vi "Wait for Return Message on FIFO Publisher.vi"(8 "error in (no error)":errorcluster, 9 "Timeout (ms)":u32=1000, 11 "CIFChannelMng in":refnum<class "CIFChannelMng.lvclass">) -> (0 "error out":errorcluster, 1 "Timeout":bool, 2 "FIFO Publisher":T1, 3 "CIFChannelMng out":refnum<class "CIFChannelMng.lvclass">)   [LabVIEW 2021, in "CIFChannelMng.lvclass"]
uses:
  CIFChannelMng.lvclass
  OOB/OOB_Tx/Typedef/FIFO Publisher Return.ctl
  typedef/Errors Channel Manager.ctl
  CIFChannelMng.lvclass/CIFChannelMng.ctl
  <vilib>/CIF Foundation/CIF Out of Band Commands/CIFOutOfBand.lvclass/CIFOutOfBand.ctl
  <vilib>/CIF Foundation/CIF Out of Band Commands/Read Commands.vi
  OOB/OOB_Tx/Private/Command Settings.vi
  OOB/OOB_Tx/Private/Read Payload.vi
  <vilib>/CIF Foundation/CIF Utilities/Errors/Append Error Location.vi
  <vilib>/CIF Foundation/CIF Out of Band Commands/Accessors/Read Local OOB Data.vi
  OOB/OOB_Tx/ChnMngOOB_Tx.lvclass
  C:/Program Files/National Instruments/LabVIEW 2021/vi.lib/CIF Foundation/CIF Out of Band Commands/CIFOutOfBand.lvclass
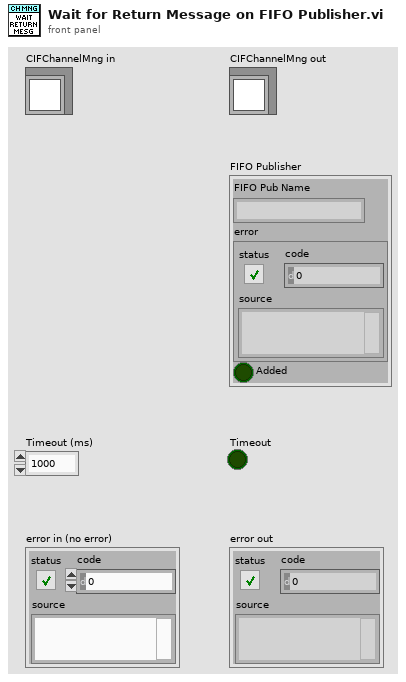
[diagram p1: front panel]
types:
  T1 = typedef "ChnMngOOB_Tx.lvclass/FIFO Publisher Return.ctl" = cluster{"FIFO Pub Name":string, "error":errorcluster, "Added":bool}
  T2 = typedef "CIFChannelMng.lvclass/Errors Channel Manager.ctl" = enum16{"gRPC Server Not Found", "Duplicate Channel", "Missing Channel", "Incorrect Type", "Flatten Error", "Unflatten Data", "Channel Length", "Plugin Connection", "gRPC Server Connection", "FIFO Unflatten", "Required Override", "Remove Not Found", "Skipped due to warning", "Timeout FIFO Pub"}
  T3 = typedef "ChnMngOOB_Tx.lvclass/OOB Core Commands.ctl" = enum8{"Channel List", "New FIFO Pub"}
  T4 = typedef "CIFChannelMng.lvclass/Channel List for OOB.ctl" = cluster{"Name":string, "Direction":T5, "Type":string, "Connected?":bool, "Connected Name":string, "Custom Config Data":u8[], "Forced?":bool, "Multi-Writer":bool}
  T5 = typedef "CIFChannels.lvclass/Direction.ctl" = enum16{"Publisher", "Subscriber"}
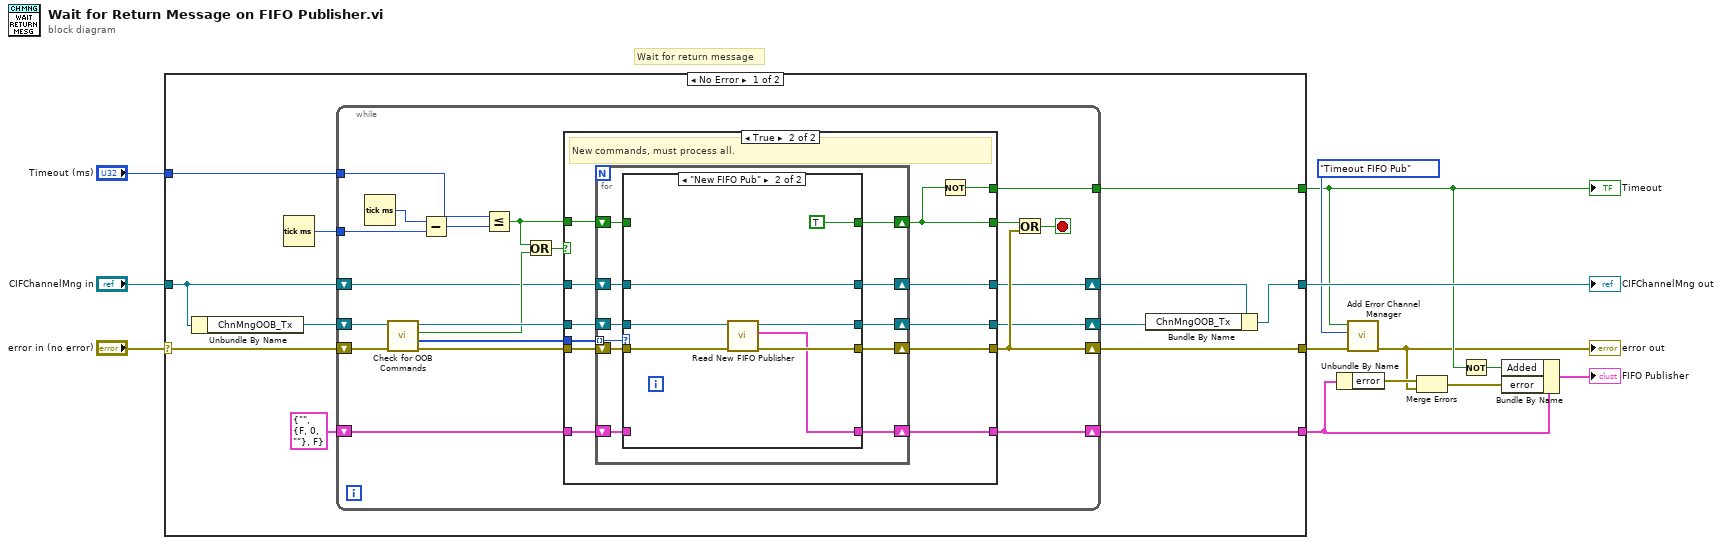
[diagram p0: block diagram]
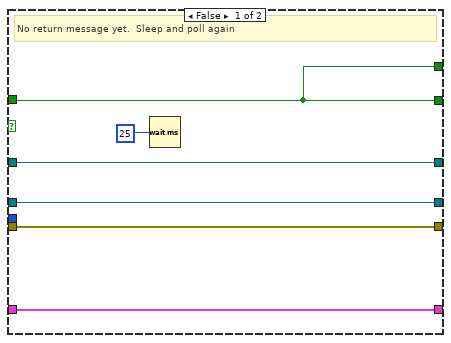
[diagram p2: hidden frame]
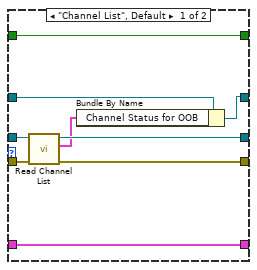
[diagram p3: hidden frame]
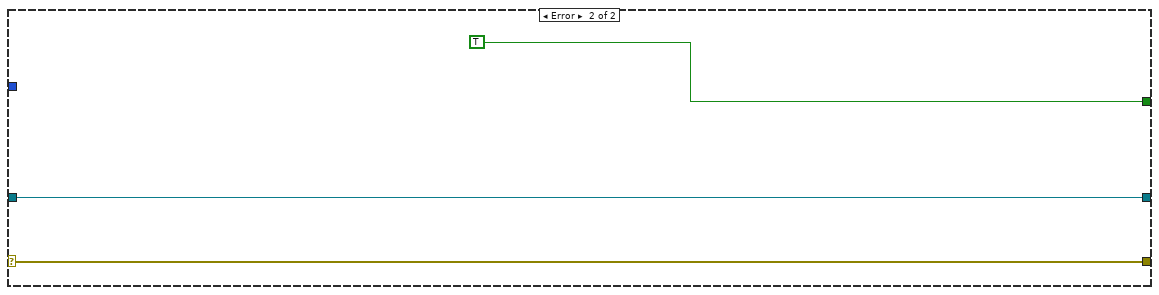
[diagram p4: hidden frame]
diagram:
  # "Wait for return message"
  n1 = case shown="No Error" "error in (no error)" {
    selector: "error in (no error)" -> [w24 w92]
    tunnel: "CIFChannelMng in" -> [w18 w93]
    tunnel: "Timeout (ms)" -> [w22 _]
    tunnel: [w21 TRUE] -> w7
    tunnel: [w20 w92] -> w9
    tunnel: [w19 _] -> w5
    tunnel: [w15 w93] -> w13
    frame No Error {
      n2 = Unbundle By Name(w18) -> ("ChnMngOOB_Tx"=w25:refnum<class "ChnMngOOB_Tx.lvclass">)
      n3 = Tick Count (ms)() -> (millisecond timer value=w23:u32)
      n4 = while {
        tunnel: w23 -> [w40]
        tunnel: w22 -> [w39]
        tunnel: [w28] -> w21
        shift-right: [w34] -> w20
        shift-left: w24 -> [w42]
        shift-right: [w31] -> w17
        shift-left: w25 -> [w46]
        shift-right: [w29] -> w16
        shift-left: w18 -> [w30]
        shift-right: [w32] -> w19
        shift-left: T1 {"FIFO Pub Name"="", "error"={"status"=FALSE, "code"=0, "source"=""}, "Added"=FALSE} ("FIFO Publisher") -> [w27]
        stop <- w33 stop-if-true
        n5 = Tick Count (ms)() -> (millisecond timer value=w41:u32)
        n6 = call "Check for OOB Commands.vi"("error in (no error)"=w42, "ChanMngOOB_Tx in"=w46) -> ("error out"=w43:errorcluster, "Commands"=w45:T3[], "New Commands"=w37:bool, "ChanMngOOB_Tx out"=w44:refnum<class "ChnMngOOB_Tx.lvclass">)  [unwired: 6 in]
        n7 = Subtract(x=w41, y=w40) -> (x-y=w38:u32)
        n8 = Less Or Equal?(x=w39, y=w38) -> (x <= y?=w26:bool)
        n9 = Or(x=w26, y=w37) -> (x .or. y?=w36:bool)
        n10 = case shown="True" w36 {
          tunnel: w45 -> [_ w64]
          tunnel: w44 -> [w50 w62]
          tunnel: w43 -> [w51 w63]
          tunnel: w26 -> [w48 w61]
          tunnel: [w48 w55] -> w35
          tunnel: [w51 w60] -> w34
          tunnel: [w47 w59] -> w32
          tunnel: [w50 w58] -> w31
          tunnel: w30 -> [w49 w57]
          tunnel: [w49 w56] -> w29
          tunnel: [w48 w54] -> w28
          tunnel: w27 -> [w47 w53]
          frame False {
            # "No return message yet.  Sleep and poll again"
            n11 = Wait (ms)(milliseconds to wait=u32 25) -> ()  [unwired: 1 out]
          }
          frame True {
            # "New commands, must process all."
            n12 = for {
              tunnel: w64 -> [w75] mode=indexing
              shift-right: [w71] -> w55
              shift-left: w61 -> [w72]
              shift-right: [w70] -> w60
              shift-left: w63 -> [w74]
              shift-right: [w68] -> w58
              shift-left: w62 -> [w73]
              shift-right: [w66] -> w56
              shift-left: w57 -> [w67]
              shift-right: [w69] -> w59
              shift-left: w53 -> [w65]
              n13 = case shown="\"New FIFO Pub\"" w75 {
                tunnel: w74 -> [w83 w89]
                tunnel: w73 -> [w84 w90]
                tunnel: w72 -> [w81 _]
                tunnel: [w81 TRUE] -> w71
                tunnel: [w82 w88] -> w70
                tunnel: [w76 w87] -> w69
                tunnel: [w80 w86] -> w68
                tunnel: [w77 w85] -> w66
                tunnel: w67 -> [w79 w85]
                tunnel: w65 -> [w76 _]
                frame "Channel List", Default {
                  n14 = call "Read Channel List.vi"("error in"=w83, "ChanMngOOB_Tx in"=w84) -> ("error out"=w82:errorcluster, "Channel List"=w78:T4[], "ChanMngOOB_Tx out"=w80:refnum<class "ChnMngOOB_Tx.lvclass">)  [unwired: 7 in]
                  n15 = Bundle By Name(cluster=w79, "Channel Status for OOB"=w78) -> (w77:refnum<class "CIFChannelMng.lvclass">)
                }
                frame "New FIFO Pub" {
                  n16 = call "Read New FIFO Publisher.vi"("error in"=w89, "ChanMngOOB_Tx in"=w90) -> ("error out"=w88:errorcluster, "FIFO Publisher"=w87:T1, "ChanMngOOB_Tx out"=w86:refnum<class "ChnMngOOB_Tx.lvclass">)  [unwired: 7 in]
                }
              }
            }
            n17 = Not(x=w55) -> (.not. x?=w54:bool)
          }
        }
        n18 = Or(x=w35, y=w34) -> (x .or. y?=w33:bool)
      }
      n19 = Bundle By Name(cluster=w16, "ChnMngOOB_Tx"=w17) -> (w15:refnum<class "CIFChannelMng.lvclass">)
    }
    frame Error {
    }
  }
  "CIFChannelMng out" <- w13
  "Timeout" <- w7
  n20 = Unbundle By Name(w5) -> ("error"=w4:errorcluster)
  n21 = call "Add Error Channel Manager.vi"("error in (no error)"=w9, "Error"=Errors_Channel_Manager."Timeout FIFO Pub", "Insert Error"=w7) -> ("error out"=w3:errorcluster)  [unwired: 8 in]
  "error out" <- w3
  n22 = Merge Errors(w4, w3) -> (w2:errorcluster)
  n23 = Not(x=w7) -> (.not. x?=w1:bool)
  n24 = Bundle By Name(cluster=w5, "Added"=w1, "error"=w2) -> (→"FIFO Publisher":T1)
